vi "tb_FIFO Empty.vi"(9 "fifo depth":u8(ring)=10 items=["4"=2, "8"=3, "16"=4, "32"=5, "64"=6, "128"=7, "256"=8, "512"=9, "1024"=10, "2048"=11, "4096"=12, "8192"=13, "16384"=14, "32768"=15, "65536"=16, "131072"=17, "262144"=18, "524288"=19, "1048576"=20, "2097152"=21, "4194304"=22, "8388608"=23, "16777216"=24, "33554432"=25, "67108864"=26, "134217728"=27, "268435456"=28, "536870912"=29, "1073741824"=30, "2147483648"=31, "4294967296"=32], 10 "arbiter configuration":T1={"write grant time (clocks)"=100, "read grant time (clocks)"=100}, 11 "Memory":T2={"fifo1 memory"="Bank0", "fifo2 memory"="Bank1"}) -> (3 "Pass?":bool=TRUE)   [LabVIEW 2011]
uses:
  <instrlib>/RF-RIO/Memory/FPGA/Interface/Timeslot Arbiter Configuration.ctl
  Data Type (256).ctl
  <instrlib>/RF-RIO/Memory/FPGA/Memory.lvlib
panel:
  in  "Stop":bool
  out "Iteration":i32
  # "This VI tests the FIFO Empty feature of the wider FIFO\n\nSequence:\n1)Push Data to FIFO continuously 500 points\n2) Send Read Requests\n3) Issue Read Requests until Data Valid out of FIFO is 500.\nThen check if FIFO Empty is True => Pass"
  # "Debug Area"
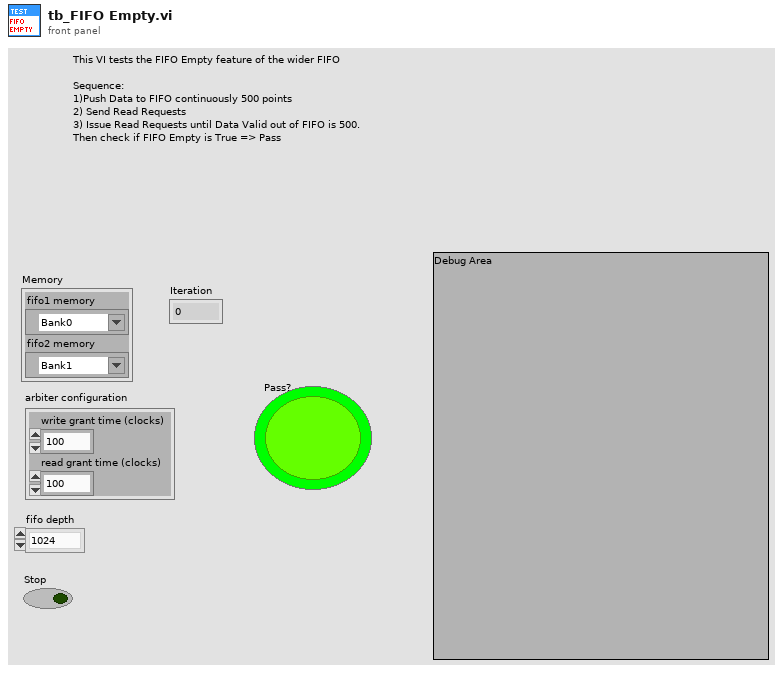
[diagram p1: front panel]
types:
  T1 = typedef "Memory.lvlib/Timeslot Arbiter Configuration.ctl" = cluster{"write grant time (clocks)":u16, "read grant time (clocks)":u16}
  T2 = cluster{"fifo1 memory":refnum<k21>, "fifo2 memory":refnum<k21>}
  T3 = typedef "Data Type (256).ctl" = cluster{"Bank0. High":u64, "Bank0. Low":u64, "Bank1. High":u64, "Bank1. Low":u64}
  T4 = typedef "FIFO.lvlib/FIFO State.ctl" = cluster{"write address":u32, "read address":u32, "full count":u32, "full":bool, "empty":bool, "in reset":bool}
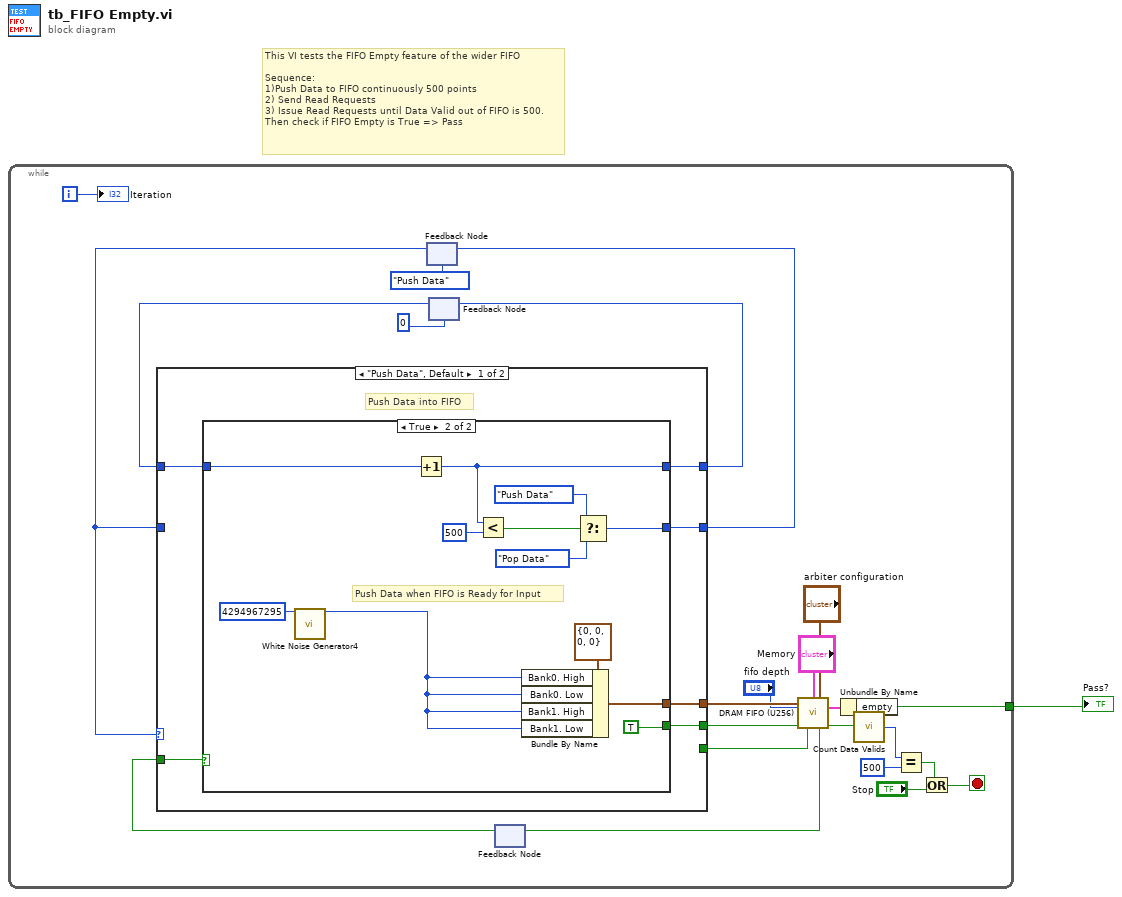
[diagram p0: block diagram]
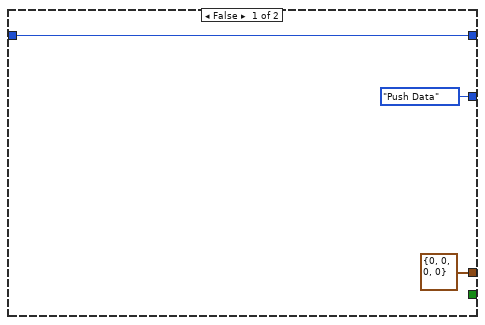
[diagram p2: hidden frame]
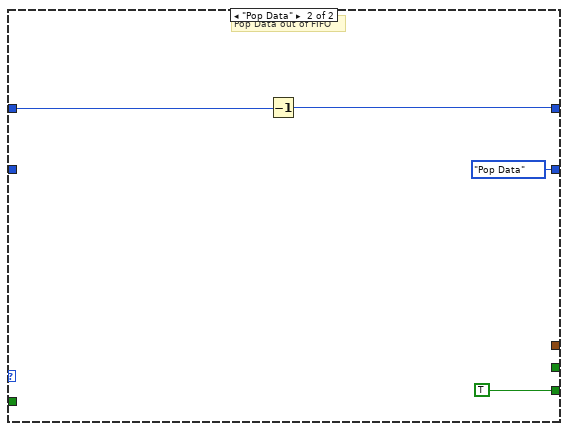
[diagram p3: hidden frame]
diagram:
  # "This VI tests the FIFO Empty feature of the wider FIFO\n\nSequence:\n1)Push Data to FIFO continuously 500 points\n2) Send Read Requests\n3) Issue Read Requests until Data Valid out of FIFO is 500.\nThen check if FIFO Empty is True => Pass"
  n1 = while {
    tunnel: [w3] -> w1
    i -> [w18]
    stop <- w5 stop-if-true
    n2 = feedback #1(enum16{"Push Data", "Pop Data", "Reset"}."Push Data") -> (w2:enum16{"Push Data", "Pop Data", "Reset"})
    n3 = feedback #2(u16 0) -> (w14:u16)
    n4 = feedback #3() -> (w22:bool)  [unwired: 1 in]
    n5 = case shown="\"Push Data\", Default" w2 {
      tunnel: [w30 _] -> w20
      tunnel: [w29 _] -> w19
      tunnel: w22 -> [w28 _]
      tunnel: [_ TRUE] -> w21
      tunnel: w14 -> [w27 w48]
      tunnel: [w26 w47] -> w15
      tunnel: [w25 enum16{"Push Data", "Pop Data", "Reset"}."Pop Data"] -> w11
      tunnel: w2 -> [_ _]
      frame "Push Data", Default {
        # "Push Data into FIFO"
        n6 = case shown="True" w28 {
          tunnel: [T3 {"Bank0. High"=0, "Bank0. Low"=0, "Bank1. High"=0, "Bank1. Low"=0} ("Input Data") w44] -> w30
          tunnel: [_ TRUE] -> w29
          tunnel: w27 -> [w32 w41]
          tunnel: [w32 w40] -> w26
          tunnel: [enum16{"Push Data", "Pop Data", "Reset"}."Push Data" w35] -> w25
          frame False {
          }
          frame True {
            # "Push Data when FIFO is Ready for Input"
            n7 = call "White Noise Generator4"("seed"=u32 4294967295) -> ("white noise out"=w34:i16)  [unwired: 14 in]
            n8 = Increment(x=w41) -> (x+1=w40:u16)
            n9 = Less?(x=w40, y=u16 500) -> (x < y?=w38:bool)
            n10 = Bundle By Name(cluster=T3 {"Bank0. High"=0, "Bank0. Low"=0, "Bank1. High"=0, "Bank1. Low"=0} ("Input Data"), "Bank0. High"=w34, "Bank0. Low"=w34, "Bank1. High"=w34, "Bank1. Low"=w34) -> (w44:T3)
            n11 = Select(t=enum16{"Push Data", "Pop Data", "Reset"}."Push Data", s=w38, f=enum16{"Push Data", "Pop Data", "Reset"}."Pop Data") -> (s? t:f=w35:enum16{"Push Data", "Pop Data", "Reset"})
          }
        }
      }
      frame "Pop Data" {
        # "Pop Data out of FIFO"
        n12 = Decrement(x=w48) -> (x-1=w47:u16)
      }
    }
    n13 = feedback-in #1(w11) -> ()
    n14 = feedback-in #2(w15) -> ()
    n15 = call "DRAM FIFO (U256).vi"("Input Data"=w20, "Memory"="Memory", "arbiter configuration"="arbiter configuration", "fifo depth"="fifo depth", "input valid"=w19, "ready for output"=w21) -> ("state"=w4:T4, "Ready for Input"=w23:bool, "Output Valid"=w10:bool)  [unwired: 4 in, 3 out]
    n16 = feedback-in #3(w23) -> ()
    n17 = Unbundle By Name(w4) -> ("empty"=w3:bool)
    n18 = call "Count Data Valids.vi"("Data Valid"=w10) -> ("Counter"=w9:u64)  [unwired: 14 in]
    n19 = Equal?(x=w9, y=u64 500) -> (x = y?=w7:bool)
    n20 = Or(x=w7, y="Stop") -> (x .or. y?=w5:bool)
    "Iteration" <- w18
  }
  "Pass?" <- w1
